vi "To Fullwidth.vi"(11 "Wide Chars":u16[](array[numeric])) -> (3 "Fullwidth Wide Chars":u16[](array[numeric]))   [LabVIEW 2020, in "G-Unicode.lvlib"]
uses:
  G-Unicode.lvlib
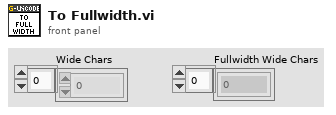
[diagram p1: front panel]
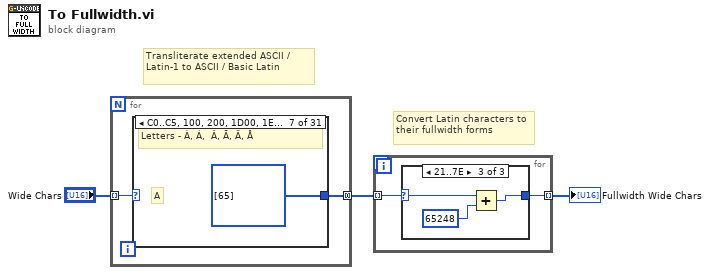
[diagram p0: block diagram]
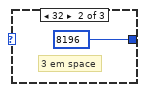
[diagram p3: hidden frame]
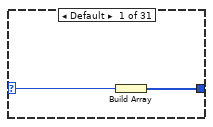
[diagram p4: hidden frame]
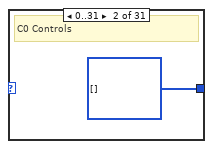
[diagram p5: hidden frame]
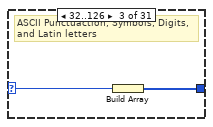
[diagram p6: hidden frame]
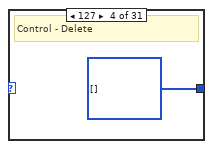
[diagram p7: hidden frame]
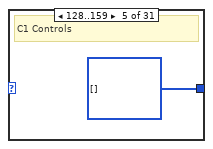
[diagram p8: hidden frame]
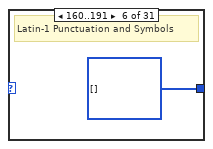
[diagram p9: hidden frame]
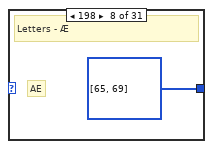
[diagram p10: hidden frame]
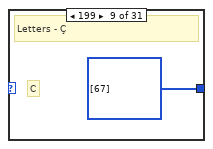
[diagram p11: hidden frame]
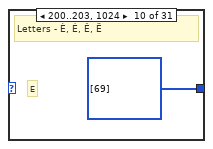
[diagram p12: hidden frame]
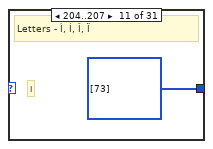
[diagram p13: hidden frame]
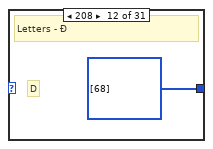
[diagram p14: hidden frame]
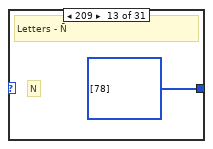
[diagram p15: hidden frame]
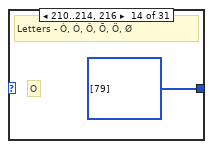
[diagram p16: hidden frame]
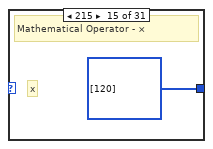
[diagram p17: hidden frame]
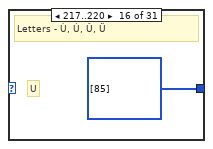
[diagram p18: hidden frame]
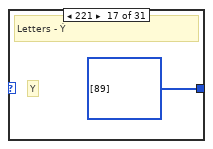
[diagram p19: hidden frame]
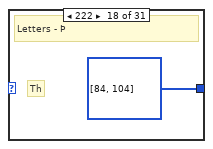
[diagram p20: hidden frame]
diagram:
  # "Convert Latin characters to their fullwidth forms"
  # "Transliterate extended ASCII / Latin-1 to ASCII / Basic Latin"
  n1 = for {
    tunnel: "Wide Chars" -> [w5] mode=indexing
    tunnel: [w4] -> w3 mode=concatenating
    n2 = case shown="C0..C5, 100, 200, 1D00, 1E00" w5 {
      selector: w5 -> [w7 _ w10 _ _ _ _ _ _ _ _ _ _ _ _ _ _ _ _ _ _ _ _ _ _ _ _ _ _ _ _]
      tunnel: [w6 u16[] [] w9 u16[] [] u16[] [] u16[] [] u16[] [65] u16[] [65, 69] u16[] [67] u16[] [69] u16[] [73] u16[] [68] u16[] [78] u16[] [79] u16[] [120] u16[] [85] u16[] [89] u16[] [84, 104] u16[] [115, 115] u16[] [97] u16[] [97, 101] u16[] [99] u16[] [101] u16[] [105] u16[] [100] u16[] [110] u16[] [111] u16[] [47] u16[] [117] u16[] [121] u16[] [116, 104]] -> w4
      frame Default {
        n3 = Build Array(w7) -> (w6:u16[])
      }
      frame 0..31 {
        # "C0 Controls"
      }
      frame 32..126 {
        # "ASCII Punctuaction, Symbols, Digits, and Latin letters"
        n4 = Build Array(w10) -> (w9:u16[])
      }
      frame 127 {
        # "Control - Delete"
      }
      frame 128..159 {
        # "C1 Controls"
      }
      frame 160..191 {
        # "Latin-1 Punctuation and Symbols"
      }
      frame 192..197, 256, 512, 7424, 7680 {
        # "A"
        # "Letters - À, Á,  Â, Ã, Ä, Å"
      }
      frame 198 {
        # "AE"
        # "Letters - Æ"
      }
      frame 199 {
        # "C"
        # "Letters - Ç"
      }
      frame 200..203, 1024 {
        # "E"
        # "Letters - È, É, Ê, Ë"
      }
      frame 204..207 {
        # "I"
        # "Letters - Ì, Í, Î, Ï"
      }
      frame 208 {
        # "D"
        # "Letters - Ð"
      }
      frame 209 {
        # "N"
        # "Letters - Ñ"
      }
      frame 210..214, 216 {
        # "O"
        # "Letters - Ò, Ó, Ô, Õ, Ö, Ø"
      }
      frame 215 {
        # "x"
        # "Mathematical Operator - ×"
      }
      frame 217..220 {
        # "U"
        # "Letters - Ù, Ú, Û, Ü"
      }
      frame 221 {
        # "Y"
        # "Letters - Ý"
      }
      frame 222 {
        # "Th"
        # "Letters - Þ"
      }
      frame 223 {
        # "ss"
        # "Letters - ß"
      }
      frame 224..229 {
        # "a"
        # "Letters - à, á,\tâ,\tã,\tä,\tå"
      }
      frame 230 {
        # "ae"
        # "Letters - æ"
      }
      frame 231 {
        # "c"
        # "Letters - ç"
      }
      frame 232..235 {
        # "e"
        # "Letters - è,\té,\tê,\të"
      }
      frame 236..239 {
        # "i"
        # "Letters - ì,\tí,\tî,\tï"
      }
      frame 240 {
        # "d"
        # "Letters - ð"
      }
      frame 241 {
        # "n"
        # "Letters - ñ"
      }
      frame 242..246, 248 {
        # "o"
        # "Letters - ò,\tó,\tô,\tõ,\tö, ø"
      }
      frame 247 {
        # "/"
        # "Letters - ÷"
      }
      frame 249..252 {
        # "u"
        # "Letters - ù,\tú,\tû,\tü"
      }
      frame 253, 255 {
        # "y"
        # "Letters - ý, ÿ"
      }
      frame 254 {
        # "th"
        # "Letters - þ"
      }
    }
  }
  n5 = for {
    tunnel: w3 -> [w40] mode=indexing
    tunnel: [w39] -> w1 mode=indexing
    n6 = case shown="21..7E" w40 {
      selector: w40 -> [w41 _ w45]
      tunnel: [w41 u16 8196 w43] -> w39
      frame Default {
      }
      frame 32 {
        # "3 em space"
      }
      frame 33..126 {
        n7 = Add(x=w45, y=u16 65248) -> (x+y=w43:u16)
      }
    }
  }
  "Fullwidth Wide Chars" <- w1
